vi "Get Tracking Test Settings.vi"(11 "Model in":refnum<class "Model.lvclass">) -> (2 "Tracking Test Settings":T1 {"Sample Time (s)" format="%.4f"; "Process Time (s)" format="%.4f"; "Repeating Error (N)" format="%.4f"}, 3 "Model out":refnum<class "Model.lvclass">)   [LabVIEW 2016, in "Model.lvclass"]
uses:
  Model.lvclass
  Typedefs/TrackingTestSettings.ctl
  Model.lvclass/Model.ctl
  Typedefs/FAMT Typedefs.lvlib
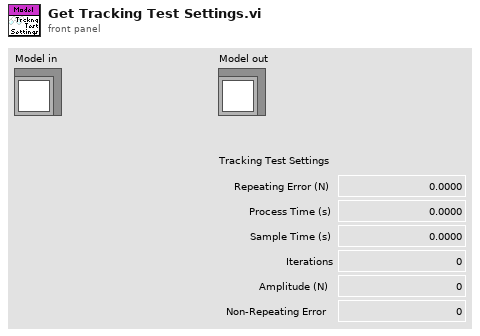
[diagram p1: front panel]
types:
  T1 = typedef "FAMT Typedefs.lvlib/TrackingTestSettings.ctl" = cluster{"Repeating Error (N)":dbl, "Process Time (s)":dbl, "Sample Time (s)":dbl, "Iterations":i32, "Amplitude (N)":dbl, "Non-Repeating Error":dbl}
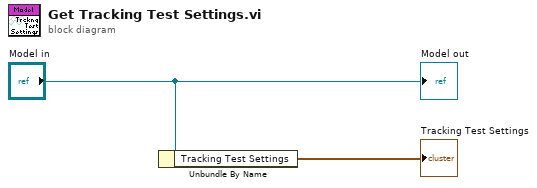
[diagram p0: block diagram]
diagram:
  n1 = Unbundle By Name("Model in") -> ("Tracking Test Settings"=→"Tracking Test Settings":T1)
  "Model out" <- "Model in"
